vi "Pockels Cal-Inner structure.vi"(1 "Index of current outer loop iteraton (Index of objective +1)":i32, 3 "Number of outer loop iteratons":i32, 5 "Objective's name":string, 9 "Number of voltage steps per objective":i32, 11 "Pockels control voltage index":i32, 12 "Pockels calibration voltage":dbl, 14 "Voltage %":u16) -> (4 "String":string, 6 "Cancel & Exit":bool, 8 "Abort this objective":bool, 10 "Timed out or errored out":bool, 15 "error out":errorcluster)   [LabVIEW 2020]
uses:
  Typedefs/Top level VI states.ctl
  Globals/gl_Calibration globals.vi
  Global Variables/gl_UI Ctrl Refs.vi
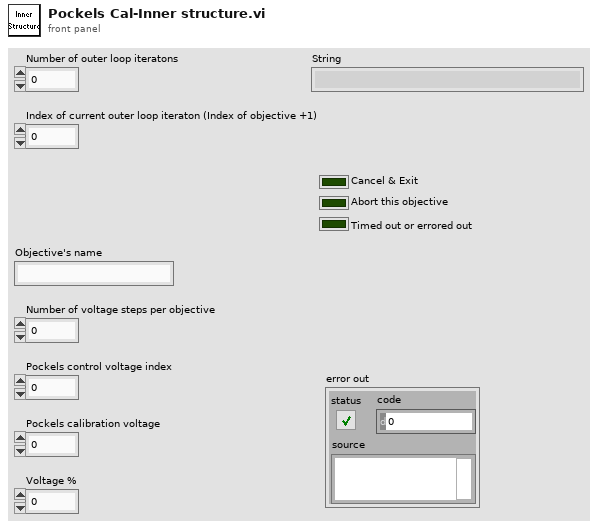
[diagram p1: front panel]
types:
  T1 = typedef "Top level VI states.ctl" = enum16{"None", "Initialise UI", "<STACK PROTOCOL STATES>", "AOL Zstack-START", "AOL Zstack-STOP", "Motor Zstack-START", "Motor Zstack-STOP", "<ACQUISITION PROTOCOL STATES> ", "Functional Acquisition-START", "Functional Acquisition-STOP", "Single Plane Acquisition-START", "Single Plane Acquisition-STOP", "Volume Acquisition-START", "Volume Acquisition-STOP", "<LIVE IMAGING PROTOCOL STATES>", "Live Imaging-START", "Live Imaging-STOP", "Live Plane Imaging-START", "Live Plane Imaging-STOP", "Live Volume Imaging-START", "Live Volume Imaging-STOP", "<MOVEMENT CORRECTION PROTOCOL STATES>", "EXIT"}
  T2 = typedef "Pockels cal process refs.ctl" = cluster{"This VI":refnum<vi>, "Abort (ind)":refnum<vi>, "Next (ind)":refnum<vi>, "Cancel":refnum<vi>, "Next":refnum<vi>, "Message":refnum<vi>, "Measured Power ctrl":refnum<vi>, "Measured Power ind":refnum<vi>, "Pockels cal progress bar":refnum<vi>, "Abort this objective":refnum<vi>}
  T3 = typedef "UI ctrl refs cluster.ctl" = cluster{"Top level VI path":path, "Top level VI ref":refnum<vi>, "User menu ref":refnum<k9>, "Sub Panel control":refnum<vi>, "Imaging Param Tab":refnum<vi>, "Occurrence-Start drivers":refnum<k4>, "Occurrence-Speed logging initialised":refnum<k4>, "Occurrence-XYZ stage initialised":refnum<k4>, "Exit button":refnum<vi>, "Status ind":refnum<vi>, "Set as origin":refnum<vi>, "Speed Logging":refnum<vi>, "Time Lapse":refnum<vi>, "Live Imaging":refnum<vi>, "AOL Z Stack":refnum<vi>, "Motor Z Stack":refnum<vi>, "Funct Acq button":refnum<vi>, "Hard Shutter":refnum<vi>, "Virtual Shutter":refnum<vi>, "Laser Power":refnum<vi>, "AOL Mode":refnum<vi>, "Frame Size":refnum<vi>, "Field of View":refnum<vi>, "Dwell Time":refnum<vi>, "Zoom":refnum<vi>, "AOL Z":refnum<vi>, "Objective":refnum<vi>, "Axis":refnum<vi>, "Paths & Names":refnum<vi>, "Experiment folder path (ind.)":refnum<vi>, "Last State (Ind.)":refnum<vi>, "Averages":refnum<vi>, "Angle (degrees)":refnum<vi>, "X centre":refnum<vi>, "Y centre":refnum<vi>, "Plane Mode":refnum<vi>, "# Planes":refnum<vi>, "Z Start":refnum<vi>, "Z Stop":refnum<vi>, "Z Step":refnum<vi>, "PMT 1":refnum<vi>, "PMT 2":refnum<vi>, "Stage XYZ Position":refnum<vi>, "Pockels@Z Start":refnum<vi>, "Pockels@Z Stop":refnum<vi>, "Obtain Z Start":refnum<vi>, "Obtain Z Stop":refnum<vi>, "Live stim.trig.period":refnum<vi>, "Live stim.trig.enable":refnum<vi>, "Movement Correction":refnum<vi>, "Load Reference Image":refnum<vi>, "XY Stage Move":refnum<vi>, "MovCor Cluster":refnum<vi>, "RefDAQParam":refnum<vi>, "Funct. Acq. Pockels Modulation":refnum<vi>, "Ref Laser Power":refnum<vi>, "Enable Video Recording":refnum<vi>, "Video Record-Live Imaging":refnum<vi>, "Video Record-Funct acq":refnum<vi>, "Reference Source":refnum<vi>, "AOL Z-stack Chirps Ready (ind)":refnum<vi>, "Target time between mov.cor. ref triggers (ms)":refnum<vi>, "Funct. Acq. Ref frame save":refnum<vi>, "Tracking button":refnum<vi>, "Show ref plots window":refnum<vi>, "Center freq ind (nm)":refnum<vi>, "Pickup mode (ind)":refnum<vi>, "Logging queue (ind)":refnum<vi>, "Back aperture power (ind.)":refnum<vi>, "Power after objective (ind.)":refnum<vi>, "Switch user":refnum<vi>, "Ls1 Conn. Status":refnum<vi>, "Ls1Tuning Status":refnum<vi>, "Ls1 Faults":refnum<vi>, "Ls1 Connection":refnum<vi>, "Ls1 Mode":refnum<vi>, "Ls1 POWER [mW]":refnum<vi>, "Ls1Shutter":refnum<vi>, "Ls1 Wavelength":refnum<vi>, "Ls1 Note":refnum<vi>, "Ls1 Confirm Wav":refnum<vi>, "Ls1 PreChrp Prism1":refnum<vi>, "Ls1 PreChrp Prism2":refnum<vi>, "Ls1 wav top Ind":refnum<vi>, "Ls1 power top Ind":refnum<vi>, "Ls1 Pump peak Hold":refnum<vi>, "Ls1 Status Ind":refnum<vi>, "Ls1 wav cancel":refnum<vi>, "Experiment Type":refnum<vi>, "Biology Information":refnum<vi>, "Camera recording status":refnum<vi>}
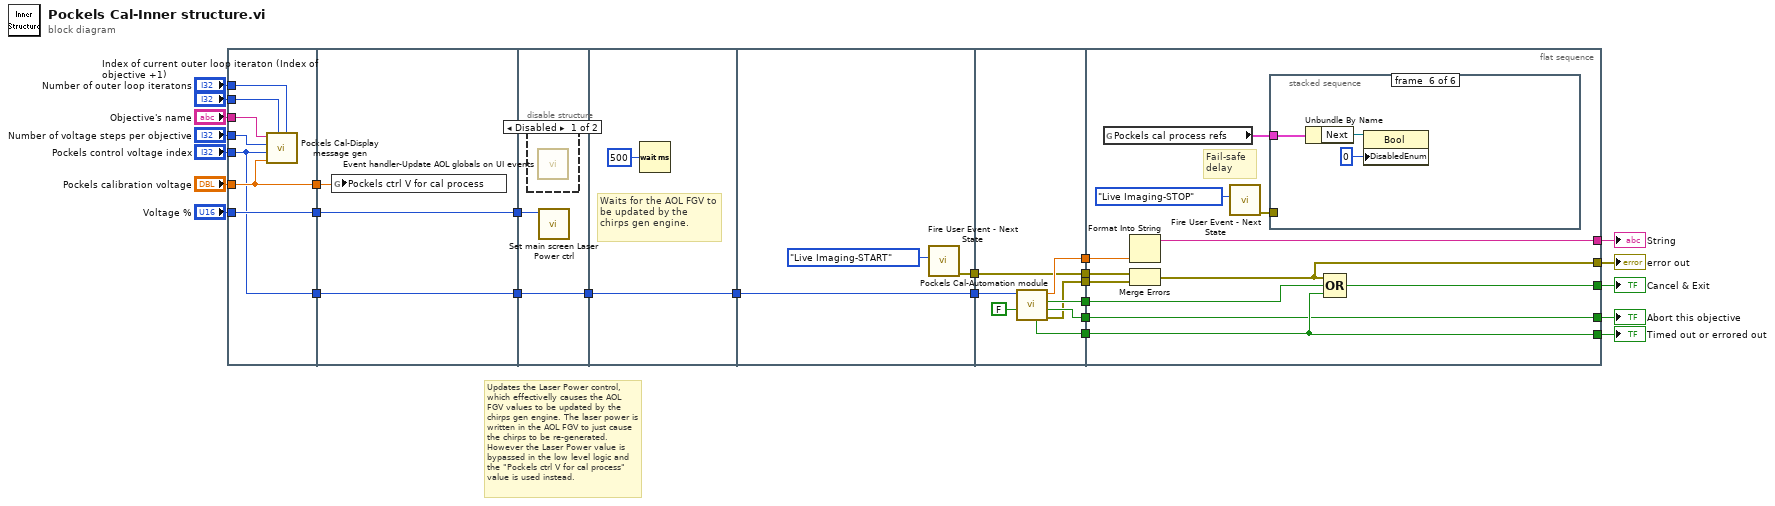
[diagram p0: block diagram]
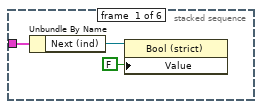
[diagram p3: hidden frame]
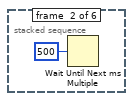
[diagram p4: hidden frame]
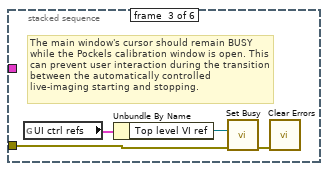
[diagram p5: hidden frame]
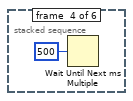
[diagram p6: hidden frame]
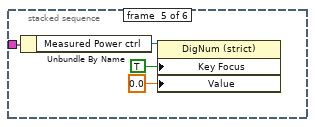
[diagram p7: hidden frame]
diagram:
  # "Updates the Laser Power control, which effectivelly causes the AOL FGV values to be updated by the chirps gen engine. The laser power is written in the AOL FGV to just cause the chirps to be re-generated. However the Laser Power value is bypassed in the low level logic and the \"Pockels ctrl V for cal process\" value is used instead."
  n1 = flat-sequence {
    tunnel: "Voltage %" -> [w34]
    tunnel: "Pockels calibration voltage" -> [w29]
    tunnel: [w29] -> w16
    tunnel: [w34] -> w15
    tunnel: "Number of outer loop iteratons" -> [w33]
    tunnel: "Index of current outer loop iteraton (Index of objective +1)" -> [w32]
    tunnel: "Objective's name" -> [w31]
    tunnel: "Number of voltage steps per objective" -> [w30]
    tunnel: "Pockels control voltage index" -> [w28]
    tunnel: [w28] -> w5
    tunnel: [w36] -> w27
    tunnel: w16 -> [w37]
    tunnel: w15 -> [w36]
    tunnel: w5 -> [w35]
    tunnel: [w35] -> w4
    tunnel: w27 -> [w39]
    tunnel: w4 -> [w38]
    tunnel: [w38] -> w3
    tunnel: w3 -> [w40]
    tunnel: [w40] -> w2
    tunnel: [w44] -> w26
    tunnel: w2 -> [w42]
    tunnel: [w42] -> w1
    tunnel: [w52] -> w25
    tunnel: [w47] -> w24
    tunnel: [w51] -> w23
    tunnel: [w50] -> w22
    tunnel: w26 -> [w50]
    tunnel: [w48] -> w7
    tunnel: [w46] -> w6
    tunnel: w1 -> [w45]
    tunnel: w25 -> [w64]
    tunnel: w24 -> [w63]
    tunnel: [w63] -> w18
    tunnel: [w62] -> w17
    tunnel: w23 -> [w59]
    tunnel: w22 -> [w55]
    tunnel: [w54] -> w19
    tunnel: [w58] -> w21
    tunnel: [w56] -> w8
    tunnel: w7 -> [w56]
    tunnel: w6 -> [w53]
    frame #0 {
      n2 = call "Pockels Cal-Display message gen.vi"("Number of outer loop iteratons"=w33, "Index of current outer loop iteraton"=w32, "Pockels control voltage"=w29, "Index of current voltage step"=w28, "Number of voltage steps per objective"=w30, "Objective name string"=w31) -> ()  [unwired: 5 in, 1 out]
    }
    frame #1 {
      n3 = global write "gl_Calibration globals.vi" "Pockels ctrl V for cal process"(w37) -> ()
    }
    frame #2 {
      n4 = disable-structure shown="Disabled" {
        frame Disabled {
          n5 = call "Event handler-Update AOL globals on UI events.vi"() -> ()  [unwired: 11 in, 1 out]
        }
        frame Enabled {
        }
      }
      n6 = call "Set main screen Laser Power ctrl.vi"("Value (Signaling)"=w39) -> ()  [unwired: 10 in, 1 out]
    }
    frame #3 {
      # "Waits for the AOL FGV to be updated by the chirps gen engine."
      n7 = Wait (ms)(milliseconds to wait=u32 500) -> ()  [unwired: 1 out]
    }
    frame #4 {
      n8 = call "Fire User Event - Next State.vi"("\"UI Handler loop\" case to execute"=Top_level_VI_states."Live Imaging-START" ("\"UI Handler loop\" case to execute")) -> ("Error Out"=w44:errorcluster)  [unwired: 10 in]
    }
    frame #5 {
      n9 = call "Pockels Cal-Automation module.vi"("Timed out"=FALSE ("Timed out while waiting for acknowledgement in"), "Pockels control voltage index"=w45) -> ("error out"=w46:errorcluster, "Abort this objective"=w48:bool, "Cancelled"=w52:bool, "Measured power"=w51:dbl, "Timed out or errored out"=w47:bool)  [unwired: 5 in]
    }
    frame #6 {
      # "Fail-safe delay"
      n10 = global read "gl_Calibration globals.vi" "Pockels cal process refs"() -> (w57:T2)
      n11 = Format Into String(w59) -> (resulting string=w58:string)  [unwired: 3 in, 1 out]
      n12 = Merge Errors(w55, w53) -> (w54:errorcluster)
      n13 = call "Fire User Event - Next State.vi"("\"UI Handler loop\" case to execute"=Top_level_VI_states."Live Imaging-STOP" ("\"UI Handler loop\" case to execute")) -> ("Error Out"=w61:errorcluster)  [unwired: 10 in]
      n14 = stacked-sequence {
        tunnel: w61 -> [_ _ w72 _ _ _]
        tunnel: w57 -> [w66 _ _ _ w74 w78]
        frame #0 {
          n15 = Unbundle By Name(w66) -> ("Next (ind)"=w65:refnum<vi>)
          n16 = property class="Bool (strict)"(reference=w65, "Value"=FALSE ("Next (ind)")) -> ()  [unwired: 1 in, 2 out]
        }
        frame #1 {
          n17 = Wait Until Next ms Multiple(millisecond multiple=u32 500 ("Delay")) -> ()  [unwired: 1 out]
        }
        frame #2 {
          # "The main window's cursor should remain BUSY while the Pockels calibration window is open. This can prevent user interaction during the transition between the automatically controlled live-imaging starting and stopping."
          n18 = global read "gl_UI Ctrl Refs.vi" "UI ctrl refs"() -> (w70:T3)
          n19 = Unbundle By Name(w70) -> ("Top level VI ref"=w69:refnum<vi>)
          n20 = call <vilib>:"Set Busy.vi"("error in (no error)"=w72, "VI reference (current VI)"=w69) -> ("error out"=w71:errorcluster)  [unwired: 8 in, 1 out]
          n21 = call <vilib>:"Clear Errors.vi"("error in (no error)"=w71) -> ()  [unwired: 5 in, 2 out]
        }
        frame #3 {
          n22 = Wait Until Next ms Multiple(millisecond multiple=u32 500 ("Delay")) -> ()  [unwired: 1 out]
        }
        frame #4 {
          n23 = Unbundle By Name(w74) -> ("Measured Power ctrl"=w75:refnum<vi>)
          n24 = property on="Property Node" class="DigNum (strict)"(reference=w75, "Key Focus"=TRUE, "Value"=0.0 ("Measured Power")) -> ()  [unwired: 1 in, 2 out]
        }
        frame #5 {
          n25 = Unbundle By Name(w78) -> ("Next"=w79:refnum<vi>)
          n26 = property on="Property Node" class="Bool"(reference=w79, "DisabledEnum"=0) -> ()  [unwired: 1 in, 2 out]
        }
      }
      n27 = Compound Arithmetic op=OR(w54, w64, w63) -> (w62:bool)
    }
  }
  "String" <- w21
  "error out" <- w19
  "Timed out or errored out" <- w18
  "Cancel & Exit" <- w17
  "Abort this objective" <- w8
